vi "Get Maximum Filename Length.vi"(8 "error in (no error)":errorcluster, 11 "Filesystem Statistics in":refnum<class "Filesystem Statistics.lvclass">) -> (0 "error out":errorcluster, 2 "maximum filename length":u64, 3 "Filesystem Statistics out":refnum<class "Filesystem Statistics.lvclass">)   [LabVIEW 2020, in "NI_SFTP.lvlib" / "Filesystem Statistics.lvclass"]
doc: "Reads the maximum filename length stored in this Filesystem Statistics object.\n\nThis property may not be supported by all servers. Additionally, it may refer to the maximum length of the entire path on some servers, but only the filename on others."
uses:
  <vilib>/net/SFTP/Filesystem Statistics/Filesystem Statistics.lvclass
  <vilib>/net/SFTP/Filesystem Statistics/Filesystem Statistics.lvclass/Filesystem Statistics.ctl
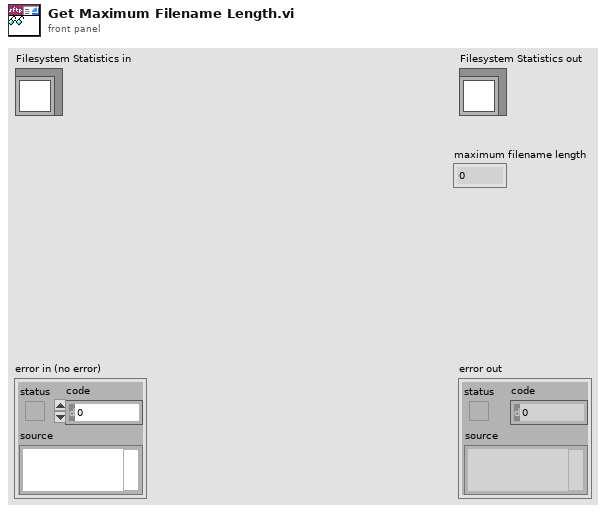
[diagram p1: front panel]
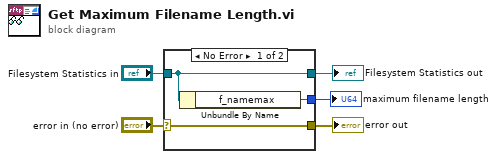
[diagram p0: block diagram]
diagram:
  n1 = case shown="No Error" "error in (no error)" {
    selector: "error in (no error)" -> [w8 w9]
    tunnel: [w8 w9] -> w4
    tunnel: [w7 w10] -> w2
    tunnel: "Filesystem Statistics in" -> [w7 w10]
    tunnel: [w6 _] -> w1
    frame No Error {
      n2 = Unbundle By Name(w7) -> ("f_namemax"=w6:u64)
    }
    frame Error {
    }
  }
  "error out" <- w4
  "Filesystem Statistics out" <- w2
  "maximum filename length" <- w1
